vi "DIO Write.vi"(1 "Data":bool[](array[boolean]), 2 "Channels":i32[](array[numeric]), 3 "device":i16=1) -> (0 "Error":bool)   [LabVIEW 2010]
uses:
  <vilib>/DAQmx/write.llb/DAQmx Write (Digital 1D Bool 1Chan 1Samp).vi
  <vilib>/DAQmx/create/channels.llb/DAQmx Create Channel (DO-Digital Output).vi
  <vilib>/daqmx/miscellaneous.llb/DAQmx Fill In Error Info.vi
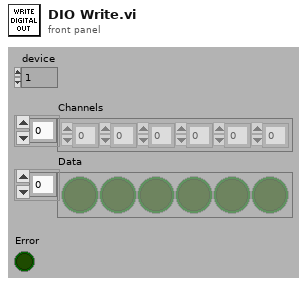
[diagram p1: front panel]
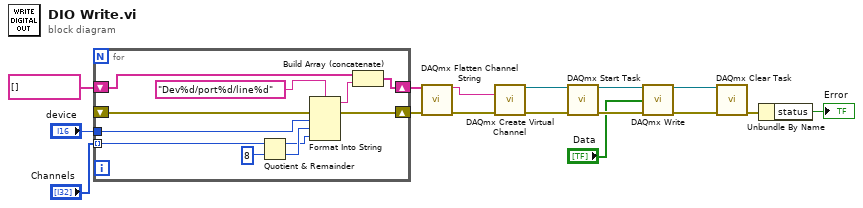
[diagram p0: block diagram]
diagram:
  n1 = for {
    tunnel: "Channels" -> [w21] mode=indexing
    tunnel: "device" -> [w20]
    shift-right: [w27] -> w15
    shift-left: tag[] [] -> [w26]
    shift-right: [w18] -> w1
    shift-left: _ -> [w17]
    n2 = Quotient & Remainder(x=w21, y=8) -> (x-y*floor(x/y)=w23:i32, floor(x/y)=w24:i32)
    n3 = Format Into String(format string="Dev%d/port%d/line%d", error in=w17, w20, w24, w23) -> (resulting string=w19:string, error out=w18:errorcluster)  [unwired: 1 in]
    n4 = Build Array (concatenate)(w26, w19) -> (w27:string[])
  }
  n5 = call <vilib>:"DAQmx Flatten Channel String.vi"("names in"=w15, "error in"=w1) -> ("names out"=w14:string, "error out"=w16:errorcluster)  [unwired: 12 in]
  n6 = call-poly <vilib>:"DAQmx Create Virtual Channel.vi"("lines"=w14, "error in"=w16) -> ("task out"=w13:refnum<k21>, "error out"=w12:errorcluster)  [unwired: 12 in]
  n7 = call <vilib>:"DAQmx Start Task.vi"("task/channels in"=w13, "error in"=w12) -> ("task out"=w11:refnum<k21>, "error out"=w10:errorcluster)  [unwired: 12 in]
  n8 = call-poly <vilib>:"DAQmx Write.vi"("task/channels in"=w11, "data"="Data", "error in"=w10) -> ("task out"=w9:refnum<k21>, "error out"=w8:errorcluster)  [unwired: 10 in, 1 out]
  n9 = call <vilib>:"DAQmx Clear Task.vi"("task in"=w9, "error in"=w8) -> ("error out"=w7:errorcluster)  [unwired: 13 in]
  n10 = Unbundle By Name(w7) -> ("status"=→"Error":bool)
